vi "Create PathMessage.vi"(8 "error in (no error)":errorcluster, 10 "Message Data":path, 11 "Message Name":string) -> (0 "error out":errorcluster, 3 "PathMsg out":refnum<class "PathMessage.lvclass">)   [LabVIEW 2009, in "LapDog.Messaging.v2.NativeTypes.lvlib" / "PathMessage.lvclass"]
doc: "Returns a PathMessage object with the given name.\n\nThis method executes regardless of the error in state."
uses:
  PathMessage.lvclass
  PathMessage.lvclass/PathMessage.ctl
  Messaging.v2/MessageObject/Message.lvclass
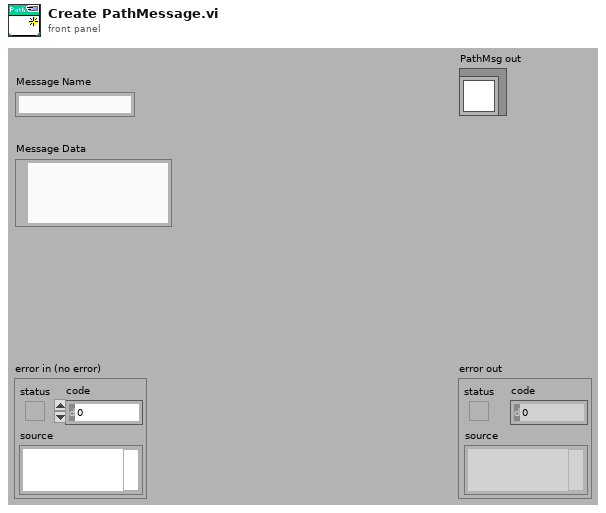
[diagram p1: front panel]
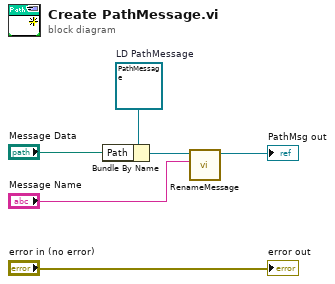
[diagram p0: block diagram]
diagram:
  w1 = refnum<class "PathMessage.lvclass"> refnum  # LD PathMessage
  n1 = Bundle By Name(cluster=w1, "Path"="Message Data") -> (w4:refnum<class "PathMessage.lvclass">)
  n2 = call "RenameMessage.vi"("Message Name"="Message Name", "Message in"=w4) -> ("Message out"=→"PathMsg out":refnum<class "PathMessage.lvclass">)  [unwired: 8 in, 1 out]
  "error out" <- "error in (no error)"
